vi "Bei Seitenwechsel abbrechen.vi"(11 "Menüstring":string) -> ()   [LabVIEW 2020, in "EPA 1065.lvlib" / "Dichtheitstest 1065-345.lvlib"]
uses:
  Dichtheitstest 1065-345.lvlib
  Aktion Leak Daten.ctl
  Aktion Leak check durchfuehren.ctl
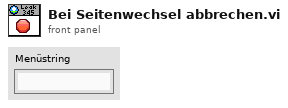
[diagram p1: front panel]
types:
  T1 = typedef "EPA 1065.lvlib/Dichtheitstest 1065-345.lvlib/Aktion Leak Daten.ctl" = enum16{"lesen", "laden", "speichern", "Volumen", "berechnen", "Leak check aktiv", "Leak Zustand", "Pfad", "Pfad speichern"}
  T2 = typedef "EPA 1065.lvlib/Dichtheitstest 1065-345.lvlib/Aktion Leak check durchfuehren.ctl" = enum16{"initialisieren", "Unterdruck erzeugen", "Ventile schließen", "Warten", "Auswertung", "fertig", "PDF erstellen", "abbrechen"}
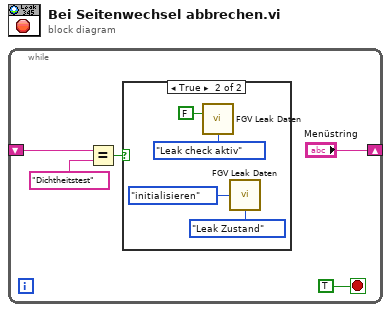
[diagram p0: block diagram]
diagram:
  n1 = while {
    shift-right: ["Menüstring"] -> _
    shift-left: _ -> [w2]
    stop <- TRUE stop-if-true
    n2 = Equal?(x=w2, y="Dichtheitstest") -> (x = y?=w1:bool)
    n3 = case shown="True" w1 {
      frame False {
      }
      frame True {
        n4 = call "FGV Leak Daten.vi"("Dichtheitstest aktiv"=FALSE, "Aktion"=Aktion_Leak_Daten."Leak check aktiv") -> ()  [unwired: 9 in, 5 out]
        n5 = call "FGV Leak Daten.vi"("Dichtheitstest Zustand"=Aktion_Leak_check_durchfuehren."initialisieren", "Aktion"=Aktion_Leak_Daten."Leak Zustand") -> ()  [unwired: 9 in, 5 out]
      }
    }
  }
